vi "Process LIDAR input.vi"(1 "Hokuyo URG Series in":refnum<class "Hokuyo URG Series.lvclass">) -> (0 "Cluster":cluster{dbl[], dbl[]})   [LabVIEW 2013]
uses:
  <instrlib>/Hokuyo URG Series/HAIOL/Hokuyo URG Series.lvclass
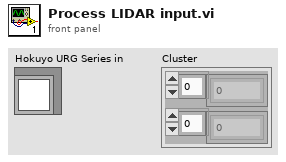
[diagram p1: front panel]
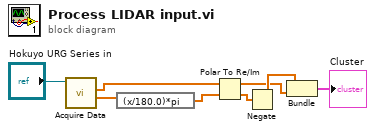
[diagram p0: block diagram]
diagram:
  n1 = call-dynamic "Acquire Data.vi"("Hokuyo URG Series in"="Hokuyo URG Series in") -> ("Direction"=w2:dbl[], "Magnitude"=w3:dbl[])  [unwired: 7 in, 2 out]
  n2 = expression code="(x/180.0)*pi" ("degrees to radians")(w2) -> (w4:dbl[])
  n3 = Polar To Re/Im(2:w4, 3:w3) -> (0:w6:dbl[], 1:w7:dbl[])
  n4 = Negate(x=w6) -> (-x=w8:dbl[])
  n5 = Bundle(w8, w7) -> (→"Cluster":cluster{dbl[], dbl[]})  [unwired: 1 in]
